vi "Angle_Calculation.vi"(0 "milliseconds to wait in":ext=1.0, 1 "Numeric in":ext, 2 "Accel Weight":dbl=0.01 format="%#_13g", 5 "LINX Resource in":T2, 7 "I2C Slave Address":T1, 9 "Offset":i16=333, 11 "error in (no error)":errorcluster, 12 "Scale_Offset":ext=2.2, 13 "Gyro_Weight":dbl=0.99 format="%#_13g") -> (3 "Accelerometer Angle Chart":dbl(graph), 4 "Numeric out":ext, 6 "Filtered Angle Chart":ext(graph)=0.14984999999999999865, 8 "Gyro Angle Chart":ext(graph)=0.15136363636363636363, 10 "milliseconds to wait out":ext, 14 "LINX Resource out":T2, 15 "error out":errorcluster)   [LabVIEW 2021]
uses:
  <vilib>/MakerHub/LINX/Private/Type Defs/LINX Ref.ctl
  <vilib>/MakerHub/LINX/Private/Type Defs/Platform.ctl
  <vilib>/MakerHub/LINX/Private/Type Defs/Interface.ctl
  <vilib>/MakerHub/LINX/Private/Device/Type Defs/LINX Device Config.ctl
  <vilib>/MakerHub/LINX/Private/Device/Type Defs/TCP Config.ctl
  <vilib>/MakerHub/LINX/Private/Device/Type Defs/Channels.ctl
  <vilib>/MakerHub/LINX/Public/Sensors/Accelerometer/MPU60X0/DeviceAddresses.ctl
  <vilib>/MakerHub/LINX/Public/Sensors/Accelerometer/MPU60X0/MPU60X0.lvlib
  <vilib>/MakerHub/LINX/LMH-LINX.lvlib
  <vilib>/MakerHub/LINX/Private/Device/Device.lvlib
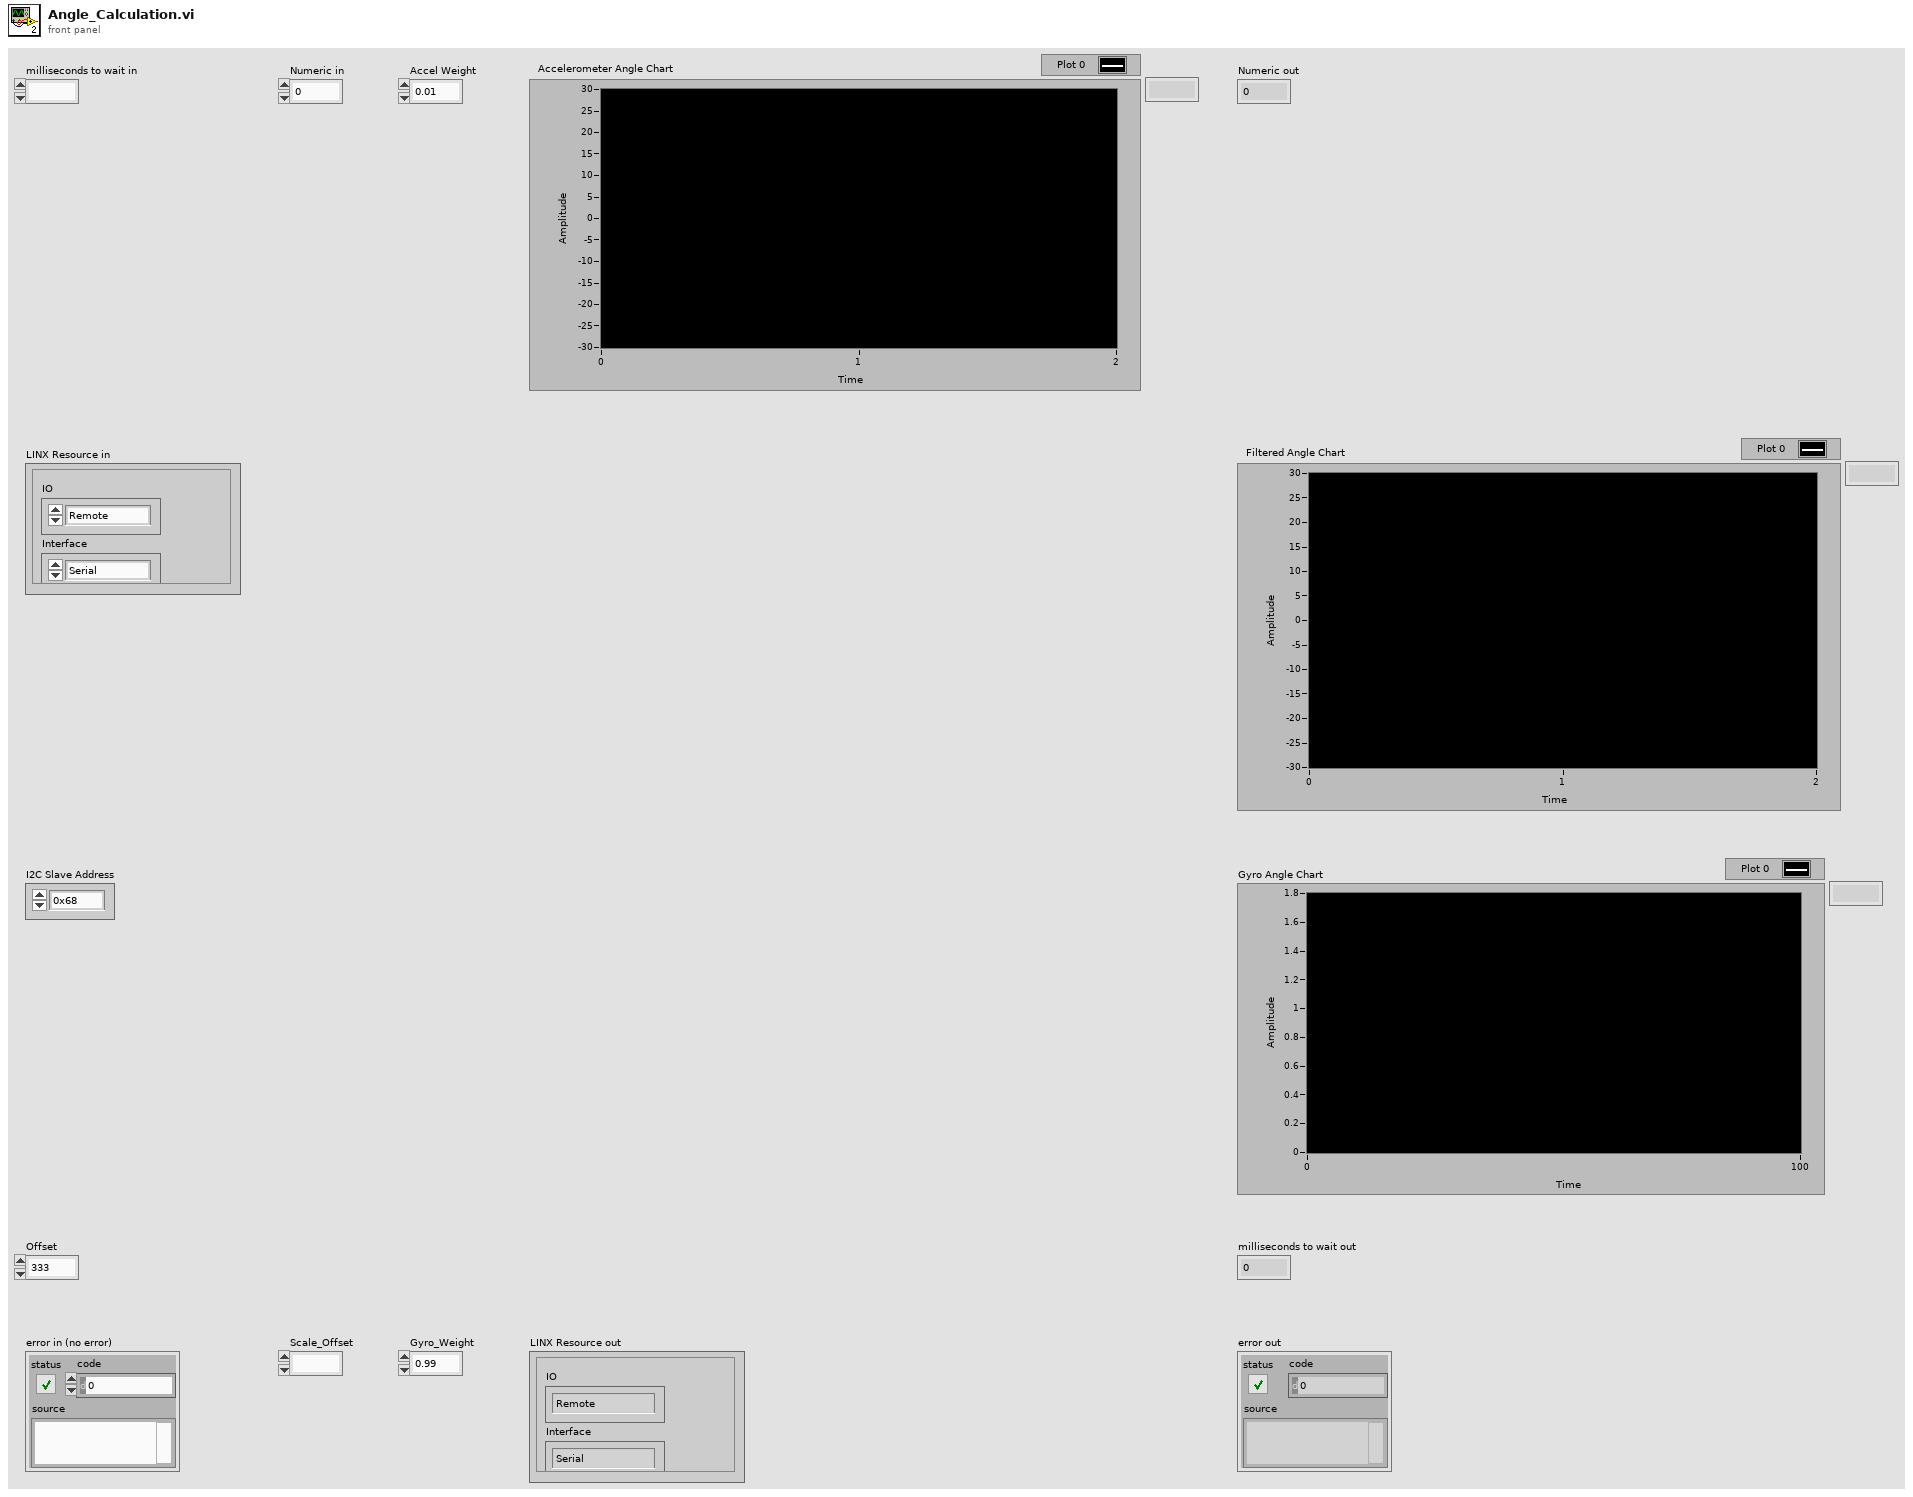
[diagram p1: front panel]
types:
  T1 = typedef "LMH-LINX.lvlib/MPU60X0.lvlib/DeviceAddresses.ctl" = enum16{"0x68", "0x69"}
  T2 = typedef "LMH-LINX.lvlib/LINX Ref.ctl" = cluster{"IO":T3, "Interface":T4, "LINX Device Config":T5}
  T3 = typedef "LMH-LINX.lvlib/Platform.ctl" = enum16{"Remote", "Local"}
  T4 = typedef "LMH-LINX.lvlib/Interface.ctl" = enum16{"Serial", "TCP"}
  T5 = typedef "LMH-LINX.lvlib/Device.lvlib/LINX Device Config.ctl" = cluster{"Interface":T4, "COM Port":refnum<visa-resource-name>, "TCP Configuration":T6, "Device Family":u8, "Device ID":u8, "Device Name":string, "TCP Ref":refnum<k5>, "Channels":T7}
  T6 = typedef "LMH-LINX.lvlib/Device.lvlib/TCP Config.ctl" = cluster{"IP Address":string, "Port":u16}
  T7 = typedef "LMH-LINX.lvlib/Channels.ctl" = cluster{"DI":u8[], "DO":u8[], "AI":u8[], "AO":u8[], "PWM":u8[], "QE":u8[], "UART":u8[], "I2C 2":u8[], "SPI":u8[], "CAN":u8[], "Servo":u8[], "AI Ref (V)":dbl, "AI Resolution (Bits)":u8, "AO Ref (V)":dbl, "AO Resolution (Bits)":u8}
  T8 = cluster{"X Axis":i16, "Y Axis":i16, "Z Axis":i16}
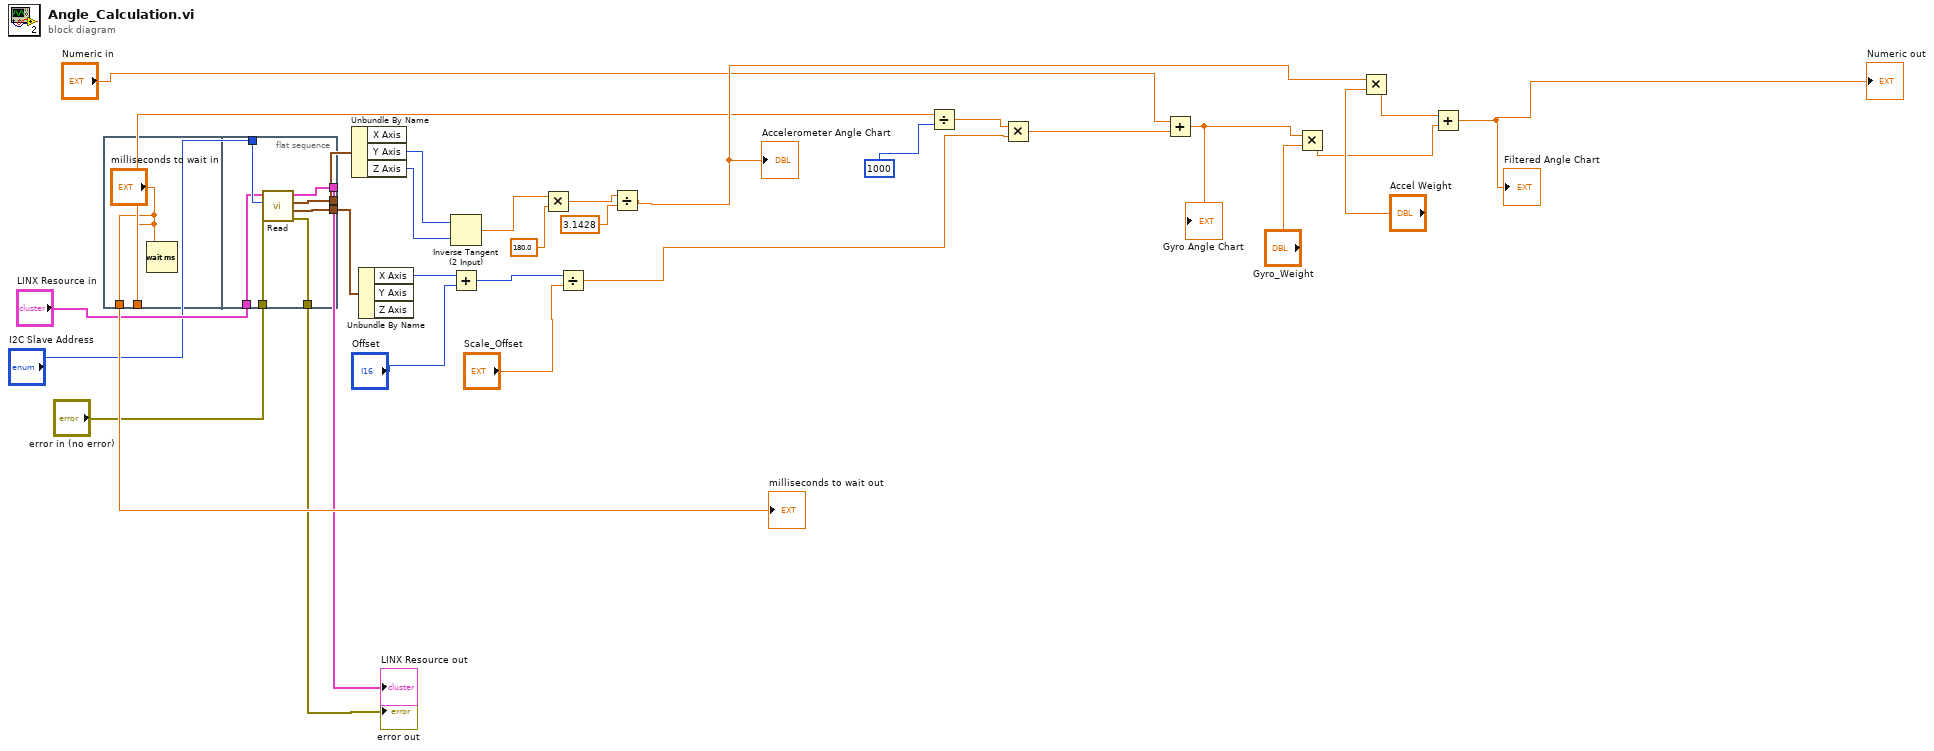
[diagram p0: block diagram]
diagram:
  n1 = flat-sequence {
    tunnel: ["milliseconds to wait in"] -> w13
    tunnel: ["milliseconds to wait in"] -> w31
    tunnel: "error in (no error)" -> [w39]
    tunnel: "I2C Slave Address" -> [w38]
    tunnel: "LINX Resource in" -> [w37]
    tunnel: [w36] -> w9
    tunnel: [w35] -> w10
    tunnel: [w34] -> w11
    tunnel: [w33] -> w12
    frame #0 {
      n2 = Wait (ms)(milliseconds to wait="milliseconds to wait in") -> ()  [unwired: 1 out]
    }
    frame #1 {
      n3 = call <vilib>:"Read.vi"("Error In"=w39, "I2C Slave Address"=w38, "LINX Resource"=w37) -> ("Error Out"=w36:errorcluster, "Gyro  Data (dps)"=w35:T8, "Acceleration Data (g)"=w34:T8, "LINX Resource"=w33:T2)  [unwired: 4 in, 1 out]
    }
  }
  n4 = Unbundle By Name(w11) -> ("Y Axis"=w20:i16, "Z Axis"=w21:i16)  [unwired: 1 out]
  n5 = Unbundle By Name(w10) -> ("X Axis"=w1:i16)  [unwired: 2 out]
  n6 = Inverse Tangent (2 Input)(1:w21, 2:w20) -> (0:w16:dbl)
  n7 = Add(x=w1, y="Offset") -> (x+y=w2:i16)
  n8 = Multiply(x=w16, y=180.0) -> (x*y=w18:dbl)
  n9 = Divide(x=w2, y="Scale_Offset") -> (x/y=w27:ext)
  n10 = Divide(x=w18, y=3.1428) -> (x/y=w22:dbl)
  "Accelerometer Angle Chart" <- w22
  n11 = Divide(x=w13, y=u32 1000) -> (x/y=w26:ext)
  n12 = Multiply(x=w26, y=w27) -> (x*y=w5:ext)
  n13 = Add(x="Numeric in", y=w5) -> (x+y=w28:ext)
  "Gyro Angle Chart" <- w28
  n14 = Multiply(x=w28, y="Gyro_Weight") -> (x*y=w23:ext)
  n15 = Multiply(x=w22, y="Accel Weight") -> (x*y=w24:dbl)
  n16 = Add(x=w24, y=w23) -> (x+y=→"Filtered Angle Chart" →"Numeric out":ext)
  "milliseconds to wait out" <- w31
  "LINX Resource out" <- w12
  "error out" <- w9
